vi "Get Segment File Size Control Caption.vi"(11 "Segment Files By":T1) -> (3 "Segment File Size Caption":string)   [LabVIEW 2027, in "Embedded Data Logger System Explorer.lvlib"]
uses:
  Embedded Data Logger System Explorer.lvlib
  Shared/Segment Files By.ctl
  Shared/Embedded Data Logger Shared.lvlib
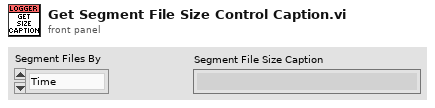
[diagram p1: front panel]
types:
  T1 = typedef "Embedded Data Logger Shared.lvlib/Segment Files By.ctl" = enum16{"Time", "Size"}
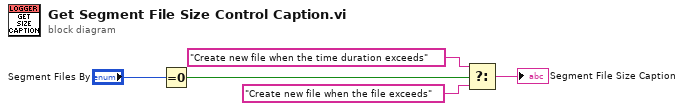
[diagram p0: block diagram]
diagram:
  n1 = Equal To 0?(x="Segment Files By") -> (x = 0?=w5:bool)
  n2 = Select(t="Create new file when the time duration exceeds" ("Caption.Text"), s=w5, f="Create new file when the file exceeds" ("Caption.Text")) -> (s? t:f=→"Segment File Size Caption":string)
